vi "labview-client.vi"() -> ()   [LabVIEW 2019]
uses:
  <vilib>/addons/zeromq/socket_type.ctl
  <vilib>/addons/zeromq/zmq_context.lvclass
  <vilib>/addons/zeromq/zmq_socket.lvclass
  <vilib>/addons/zeromq/zeromq.lvlib
panel:
  in  "TCP address":string="tcp://127.0.0.1:5555"
  in  "command":string="test()"
  out "data":string
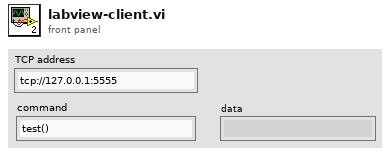
[diagram p1: front panel]
types:
  T1 = typedef "zeromq.lvlib/socket_type.ctl" = enum8{"ZMQ_PAIR", "ZMQ_PUB", "ZMQ_SUB", "ZMQ_REQ", "ZMQ_REP", "ZMQ_DEALER", "ZMQ_ROUTER", "ZMQ_PULL", "ZMQ_PUSH", "ZMQ_XPUB", "ZMQ_XSUB", "ZMQ_STREAM", "ZMQ_SERVER", "ZMQ_CLIENT", "ZMQ_RADIO", "ZMQ_DISH", "ZMQ_GATHER", "ZMQ_SCATTER", "ZMQ_DGRAM"}
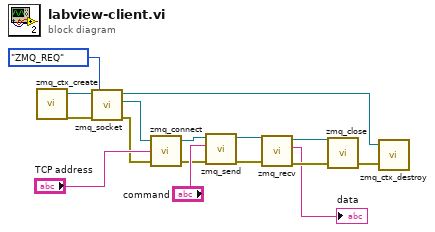
[diagram p0: block diagram]
diagram:
  n1 = call <vilib>:"zmq_ctx_create.vi"() -> ("error out"=w15:errorcluster, "context out"=w16:refnum<class "zmq_context.lvclass">)  [unwired: 4 in]
  n2 = call <vilib>:"zmq_socket.vi"("error in"=w15, "socket type"=socket_type."ZMQ_REQ", "context in"=w16) -> ("error out"=w11:errorcluster, "socket out"=w12:refnum<class "zmq_socket.lvclass">, "context out"=w3:refnum<class "zmq_context.lvclass">)  [unwired: 2 in]
  n3 = call <vilib>:"zmq_connect.vi"("error in"=w11, "endpoint"="TCP address", "socket in"=w12) -> ("error out"=w9:errorcluster, "socket out"=w8:refnum<class "zmq_socket.lvclass">)  [unwired: 1 in]
  n4 = call <vilib>:"zmq_send.vi"("error in"=w9, "data"="command", "socket in"=w8) -> ("error out"=w7:errorcluster, "socket out"=w6:refnum<class "zmq_socket.lvclass">)  [unwired: 4 in]
  n5 = call <vilib>:"zmq_recv.vi"("error in"=w7, "socket in"=w6) -> ("error out"=w5:errorcluster, "data"=→"data":string, "socket out"=w1:refnum<class "zmq_socket.lvclass">)  [unwired: 3 in, 2 out]
  n6 = call <vilib>:"zmq_close.vi"("error in"=w5, "socket"=w1) -> ("error out"=w4:errorcluster)  [unwired: 3 in]
  n7 = call <vilib>:"zmq_ctx_destroy.vi"("error in"=w4, "context in"=w3) -> ()  [unwired: 3 in, 1 out]
